vi "DCA Convert 1.3 - 1.4 to 1.8.vi"(1 "DCA 1.3 - 1.4 Test Parameters":T2={"Tag"="", "Use Instrument"=FALSE, "Quick Mode"=FALSE, "Topology"=enum."Pi", "Zo"=50.0, "Range"=0, "Resolution"=0, "Blank Screen"=FALSE, "Limits"=[], "Reports"={"Reports to Generate"=[], "Print Reports"=TRUE}, "Lock Topology"=FALSE, "Normalize"=TRUE} {"Resolution" items=["Auto", "4 1/2", "5 1/2", "6 1/2"]; "Range" items=["Auto", "Min", "Max", "100", "1,000", "10,000", "100,000", "1,000,000", "10,000,000", "100,000,000"]}) -> (0 "DCA 1.8 Test Parameters":T1={"Tag"="", "Use Instrument"=FALSE, "Quick Mode"=FALSE, "Topology"=enum."Pi", "Zo"=50.0, "Range"=0, "Resolution"=0, "Blank Screen"=FALSE, "Limits"=[], "Datasheets"={"Datasheets to Generate"=[], "Print Datasheets"=TRUE}, "Lock Topology"=FALSE, "Normalize"=TRUE, "ATTN Calc"=enum."Power"} {"Resolution" items=["Auto", "4 1/2", "5 1/2", "6 1/2"]; "Range" items=["Auto", "Min", "Max", "100", "1,000", "10,000", "100,000", "1,000,000", "10,000,000", "100,000,000"]; "Limits"."Run" min=1 step=1})   [LabVIEW 2011]
uses:
  TypeDefs/DCA Test Parameters v1.3-1.4.ctl
  TypeDefs/DCA Test Parameters v1.8.ctl
panel:
  # "="
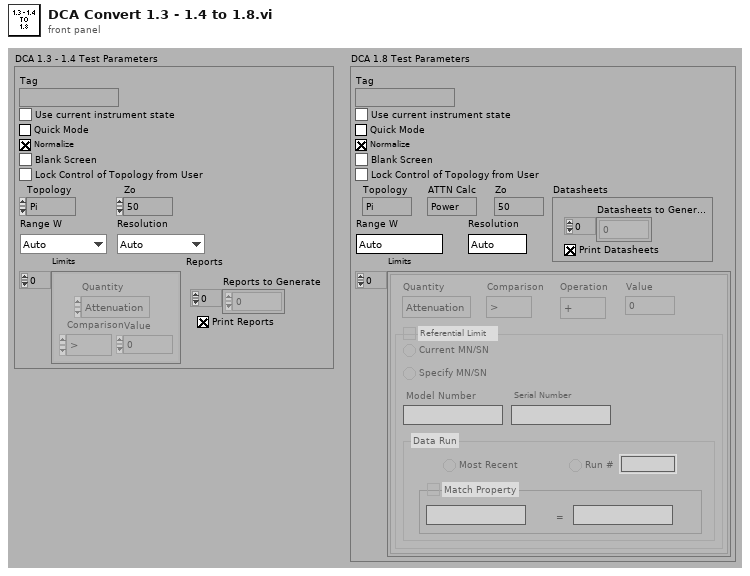
[diagram p1: front panel]
types:
  T1 = typedef "DCA Test Parameters v1.8.ctl" = cluster{"Tag":string, "Use Instrument":bool, "Quick Mode":bool, "Topology":enum32{"Pi", "T"}, "Zo":dbl, "Range":u16, "Resolution":u16, "Blank Screen":bool, "Limits":cluster{"Quantity":enum16{"Attenuation", "Zin", "Zout", "R1", "R2", "R3", "Rab", "Rac", "Rbc"}, "Comparison":enum16{">", ">=", "<", "<=", "+", "-"}, "Operation":enum16{"+", "-"}, "Value":dbl, "Ref Limit":bool, "Ref Type":enum32{"Current", "Specify"}, "Model":string, "Serial":string, "Run Type":enum32{"Most Recent", "Run #"}, "Run":i32, "Match Property":bool, "Property":string, "Property Value":string}[], "Datasheets":cluster{"Datasheets to Generate":i32[], "Print Datasheets":bool}, "Lock Topology":bool, "Normalize":bool, "ATTN Calc":enum32{"Power", "Voltage"}}
  T2 = typedef "DCA Test Parameters v1.3-1.4.ctl" = cluster{"Tag":string, "Use Instrument":bool, "Quick Mode":bool, "Topology":enum32{"Pi", "T"}, "Zo":dbl, "Range":u16, "Resolution":u16, "Blank Screen":bool, "Limits":cluster{"Quantity":enum16{"Attenuation", "Zin", "Zout", "R1", "R2", "R3", "Rab", "Rac", "Rbc"}, "Comparison":enum16{">", ">=", "<", "<="}, "Value":dbl}[], "Reports":cluster{"Reports to Generate":i32[], "Print Reports":bool}, "Lock Topology":bool, "Normalize":bool}
  T3 = cluster{"Quantity":enum16{"Attenuation", "Zin", "Zout", "R1", "R2", "R3", "Rab", "Rac", "Rbc"}, "Comparison":enum16{">", ">=", "<", "<=", "+", "-"}, "Operation":enum16{"+", "-"}, "Value":dbl, "Ref Limit":bool, "Ref Type":enum32{"Current", "Specify"}, "Model":string, "Serial":string, "Run Type":enum32{"Most Recent", "Run #"}, "Run":i32, "Match Property":bool, "Property":string, "Property Value":string}[]
  T4 = cluster{"Reports to Generate":i32[], "Print Reports":bool}
  T5 = cluster{"Quantity":enum16{"Attenuation", "Zin", "Zout", "R1", "R2", "R3", "Rab", "Rac", "Rbc"}, "Comparison":enum16{">", ">=", "<", "<="}, "Value":dbl}[]
  T6 = cluster{"Quantity":enum16{"Attenuation", "Zin", "Zout", "R1", "R2", "R3", "Rab", "Rac", "Rbc"}, "Comparison":enum16{">", ">=", "<", "<=", "+", "-"}, "Operation":enum16{"+", "-"}, "Value":dbl, "Ref Limit":bool, "Ref Type":enum32{"Current", "Specify"}, "Model":string, "Serial":string, "Run Type":enum32{"Most Recent", "Run #"}, "Run":i32, "Match Property":bool, "Property":string, "Property Value":string}
  T7 = enum16{"Attenuation", "Zin", "Zout", "R1", "R2", "R3", "Rab", "Rac", "Rbc"}
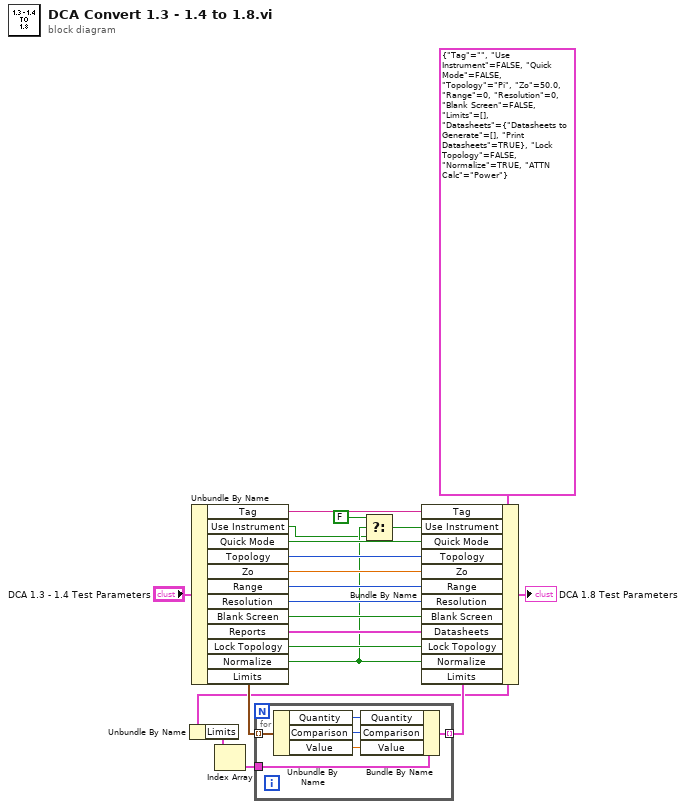
[diagram p0: block diagram]
diagram:
  w1 = T1 {"Tag"="", "Use Instrument"=FALSE, "Quick Mode"=FALSE, "Topology"=enum."Pi", "Zo"=50.0, "Range"=0, "Resolution"=0, "Blank Screen"=FALSE, "Limits"=[], "Datasheets"={"Datasheets to Generate"=[], "Print Datasheets"=TRUE}, "Lock Topology"=FALSE, "Normalize"=TRUE, "ATTN Calc"=enum."Power"} ("DCA 1.9 Test Parameters")
  n1 = Unbundle By Name(w1) -> ("Limits"=w10:T3)
  n2 = Unbundle By Name("DCA 1.3 - 1.4 Test Parameters") -> ("Tag"=w20:string, "Use Instrument"=w4:bool, "Quick Mode"=w19:bool, "Topology"=w18:enum32{"Pi", "T"}, "Zo"=w17:dbl, "Range"=w16:u16, "Resolution"=w15:u16, "Blank Screen"=w14:bool, "Reports"=w11:T4, "Lock Topology"=w13:bool, "Normalize"=w7:bool, "Limits"=w12:T5)
  n3 = Index Array(array=w10) -> (element=w9:T6)  [unwired: 1 in]
  n4 = for {
    tunnel: w12 -> [w26] mode=indexing
    tunnel: w9 -> [w25]
    tunnel: [w21] -> w8 mode=indexing
    n5 = Unbundle By Name(w26) -> ("Quantity"=w22:T7, "Comparison"=w23:enum16{">", ">=", "<", "<="}, "Value"=w24:dbl)
    n6 = Bundle By Name(cluster=w25, "Quantity"=w22, "Comparison"=w23, "Value"=w24) -> (w21:T6)
  }
  n7 = Select(t=FALSE, s=w7, f=w4) -> (s? t:f=w6:bool)
  n8 = Bundle By Name(cluster=w1, "Tag"=w20, "Use Instrument"=w6, "Quick Mode"=w19, "Topology"=w18, "Zo"=w17, "Range"=w16, "Resolution"=w15, "Blank Screen"=w14, "Datasheets"=w11, "Lock Topology"=w13, "Normalize"=w7, "Limits"=w8) -> (→"DCA 1.8 Test Parameters":T1)
